vi "Read Voltage Setpoint (Array).vi"(8 "error in":errorcluster, 11 "Voltage Control in":refnum<class "Voltage Control.lvclass">) -> (0 "error out":errorcluster, 1 "Changed or First Call?":bool, 2 "Voltage Setpoint":dbl[](array[numeric]), 3 "Voltage Control out":refnum<class "Voltage Control.lvclass">)   [LabVIEW 2023, in "Voltage Control.lvclass"]
doc: "This VI will read all setpoints for all channels"
uses:
  Voltage Control.lvclass
  Voltage Control.lvclass/Voltage Control.ctl
  <vilib>/ADAS Replay HIL/Channels/Tag Wrapper/Polymorphic/Read Channel (Double).vi
  e91dbfa7-f59d-4619-a9dc-d66410cba252.vi
  <vilib>/ADAS Replay HIL/Channels/Tag Wrapper/Polymorphic/Read Channel (Double).vi/b2f764de-0c1e-4784-a155-687fc995a684.vi
  <vilib>/ADAS Replay HIL/Channels/Tag Wrapper/Polymorphic/Read Channel (Double).vi/b2f764de-0c1e-4784-a155-687fc995a684.vi/c28b0ead-42ad-4072-80a2-aca7f2bd7ce3.vi
  <vilib>/ADAS Replay HIL/Channels/Tag Wrapper/Polymorphic/Read Channel (Double).vi/b2f764de-0c1e-4784-a155-687fc995a684.vi/219d0231-d98b-4193-b5cc-84f90e3c9091.vi
  <vilib>/ADAS Replay HIL/Channels/Tag Wrapper/Tag Wrapper.lvlib
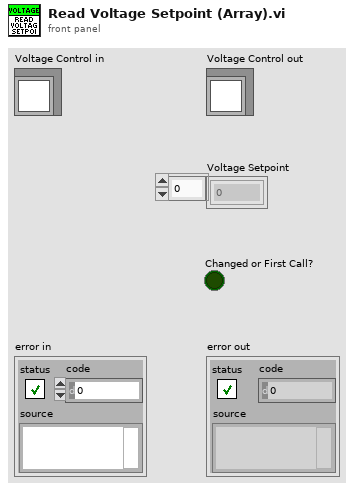
[diagram p1: front panel]
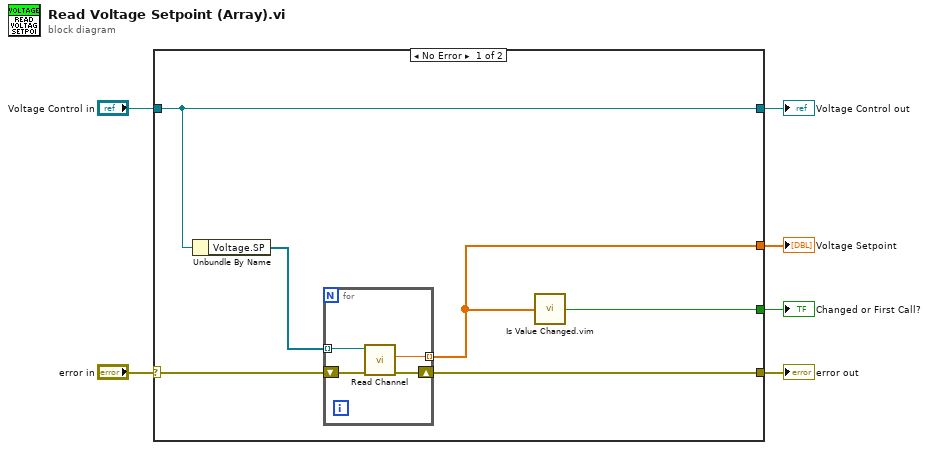
[diagram p0: block diagram]
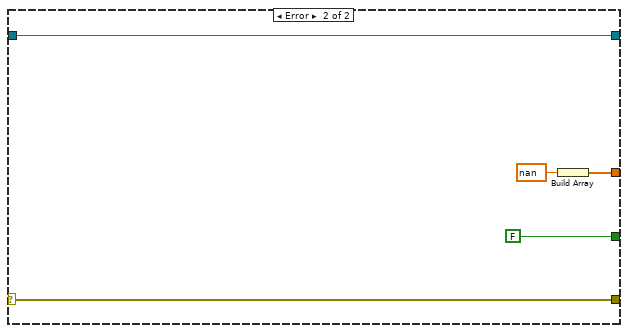
[diagram p2: hidden frame]
diagram:
  n1 = case shown="No Error" "error in" {
    selector: "error in" -> [w10 w21]
    tunnel: [w9 w21] -> w5
    tunnel: [w12 w20] -> w3
    tunnel: "Voltage Control in" -> [w12 w20]
    tunnel: [w8 w17] -> w2
    tunnel: [w7 FALSE ("changed or first call?")] -> w1
    frame No Error {
      n2 = Unbundle By Name(w12) -> ("Voltage.SP"=w11:refnum<k21>[])
      n3 = for {
        tunnel: w11 -> [w16] mode=indexing
        tunnel: [w13] -> w8 mode=indexing
        shift-right: [w14] -> w9
        shift-left: w10 -> [w15]
        n4 = call-poly <vilib>:"Read Channel.vi"("error in"=w15, "ADAS HIL Channel in"=w16) -> ("error out"=w14:errorcluster, "Value out"=w13:dbl)  [unwired: 6 in, 2 out]
      }
      n5 = call "Is Value Changed.vim"("value"=w8) -> ("changed or first call?"=w7:bool)
    }
    frame Error {
      n6 = Build Array(nan ("Value out")) -> (w17:dbl[])
    }
  }
  "error out" <- w5
  "Voltage Control out" <- w3
  "Voltage Setpoint" <- w2
  "Changed or First Call?" <- w1
